vi "InitializeSolenoid.vi"() -> (0 "error out":T1)   [LabVIEW 2014]
uses:
  ErrorOut.ctl
  <vilib>/Rock Robotics/WPI/Solenoid/WPI_SolenoidOpenDouble.vi
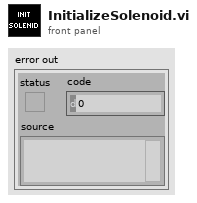
[diagram p1: front panel]
types:
  T1 = typedef "ErrorOut.ctl" = errorcluster
  T2 = typedef "WPI_SolenoidDevRef.ctl" = cluster{"DevStatus":errorcluster, "Pneumatics Control Module":u8, "Forward Solenoid Channel":T3, "Reverse Solenoid Channel":T3}
  T3 = typedef "WPI_SolenoidChannel.ctl" = enum8{"Solenoid 0", "Solenoid 1", "Solenoid 2", "Solenoid 3", "Solenoid 4", "Solenoid 5", "Solenoid 6", "Solenoid 7", "Invalid"}
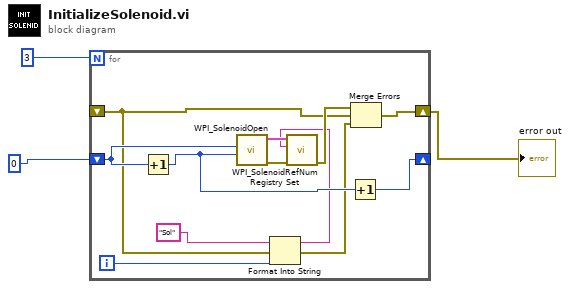
[diagram p0: block diagram]
diagram:
  n1 = for {
    N: 3 -> [_]
    shift-right: [w11] -> _
    shift-left: 0 -> [w12]
    shift-right: [w9] -> w1
    shift-left: _ -> [w7]
    i -> [w6]
    n2 = Increment(x=w12) -> (x+1=w13:i32)
    n3 = call-poly <vilib>:"WPI_SolenoidOpen.vi"("Reverse Solenoid Channel"=w13, "Forward Solenoid Channel"=w12) -> ("error out"=w15:errorcluster, "SolenoidDevRef"=w14:T2)  [unwired: 8 in]
    n4 = Format Into String(initial string="Sol", error in=w7, w6) -> (resulting string=w4:string, error out=w5:errorcluster)  [unwired: 1 in]
    n5 = call <vilib>:"WPI_SolenoidRefNum Registry Set.vi"("error in (no error)"=w15, "refnum name"=w4, "SolenoidDevRef"=w14) -> ("error out"=w10:errorcluster)  [unwired: 7 in, 1 out]
    n6 = Increment(x=w13) -> (x+1=w11:i32)
    n7 = Merge Errors(w10, w7, w5) -> (w9:errorcluster)
  }
  "error out" <- w1
